vi "Set Footers.vi"(8 "error in (no error)":errorcluster, 10 "Footers":refnum<class "xwpfFooter.lvclass">[](array[class]), 11 "xwpfDocument in":refnum<class "xwpfDocument.lvclass">) -> (0 "error out":errorcluster, 3 "xwpfDocument out":refnum<class "xwpfDocument.lvclass">)   [LabVIEW 2017, in "LabVIEW NPOI.lvlib" / "xwpfDocument.lvclass"]
uses:
  xwpfDocument.lvclass
  xwpfFooter/xwpfFooter.lvclass
  xwpfDocument.lvclass/xwpfDocument.ctl
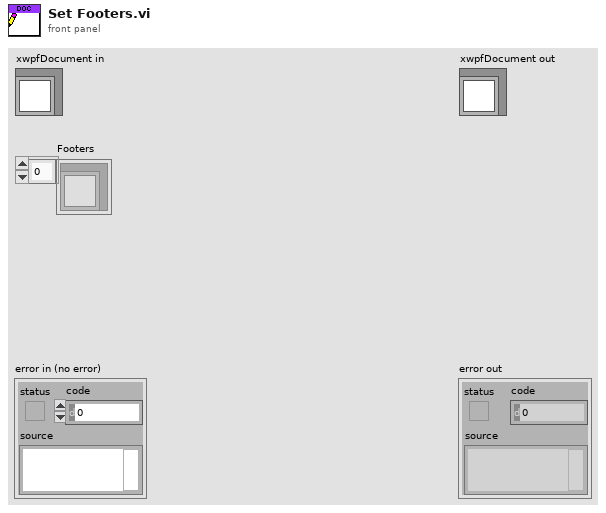
[diagram p1: front panel]
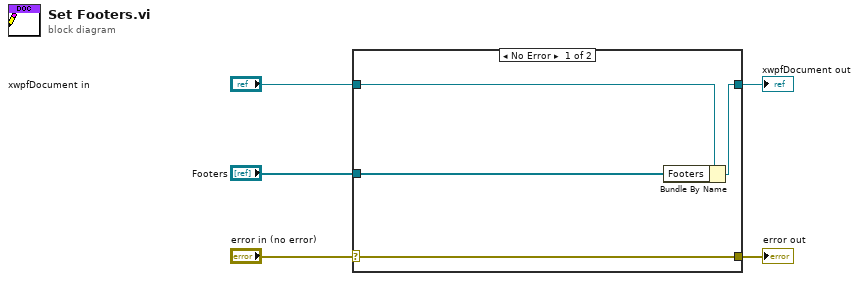
[diagram p0: block diagram]
diagram:
  n1 = case shown="No Error" "error in (no error)" {
    selector: "error in (no error)" -> [w9 w10]
    tunnel: [w9 w10] -> w4
    tunnel: [w7 w11] -> w2
    tunnel: "xwpfDocument in" -> [w8 w11]
    tunnel: "Footers" -> [w6 _]
    frame No Error {
      n2 = Bundle By Name(cluster=w8, "Footers"=w6) -> (w7:refnum<class "xwpfDocument.lvclass">)
    }
    frame Error {
    }
  }
  "error out" <- w4
  "xwpfDocument out" <- w2
